vi "ExperimentStateCluster.vi"() -> (2 "Experiment State":T1={"error"={"status"=FALSE, "code"=0, "source"=""}, "Digitizer DAQmx Tasks"={"TaskArray"=[]}, "Digitizer Settings"={"Channel Settings"=[], "Card Settings"=[]}, "Synchronization Settings"={"Synchronizer"="PXI1Slot2", "source terminal"="GlobalSoftwareTrigger"}, "Digitizer Data"=[], "Next Shot#"="0", "System Message"="", "User Shot Notes"="", "Timing Settings"={"Timing Card Settings"=[], "Timing Channel Settings"=[[{"Delay (s)"=2.559999942779541, "Pulse width (s)"=0.009999999776482582, "Active"=TRUE, "Channel Name"="Fiber 8", "counter"="PXI1Slot8/ctr7", "FrontPanelTime"=2.559999942779541}]]}, "Timing Tasks"={"TaskArray"=[]}, "Tree"="0", "Time Card/Channels"=[2, 8], "DAQ Card/Channels"=[3, 8], "Program Version"="", "RIO Settings"={"Channel Settings"=[], "Card Settings"=[]}, "RIO References"={"Reference Array"=[]}} {"RIO Settings"."Card Settings"."Sample Rate" format="%#_3p"; "Timing Settings"."Timing Channel Settings"."FrontPanelTime" format="%.3p"; "Timing Settings"."Timing Channel Settings"."Pulse width (s)" format="%.3p"; "Timing Settings"."Timing Channel Settings"."Delay (s)" format="%.3p"; "Digitizer Settings"."Card Settings"."Global Edge Type" items=["Rising"=10280, "Falling"=10171]; "Digitizer Settings"."Card Settings"."Sample Rate" format="%#_3p"})   [LabVIEW 2014]
uses:
  ExperimentStateCluster.ctl
  DigitizerSettingsChannelSettings.ctl
  DigitizerSettingsCardSettingsArray.ctl
  DigitizerSettingsCardSettings.ctl
  TimingSettings.ctl
  TimingCardSettings.ctl
  TimingChannelSettings.ctl
  RIOSettingsExperimentStateCluster.ctl
  RIOSettingsChannelSettings.ctl
  RIOSettingsCardSettingsArray.ctl
  RIOSettingsCardSettings.ctl
  <vilib>/userdefined/High Color/nirio_resource_hc.ctl
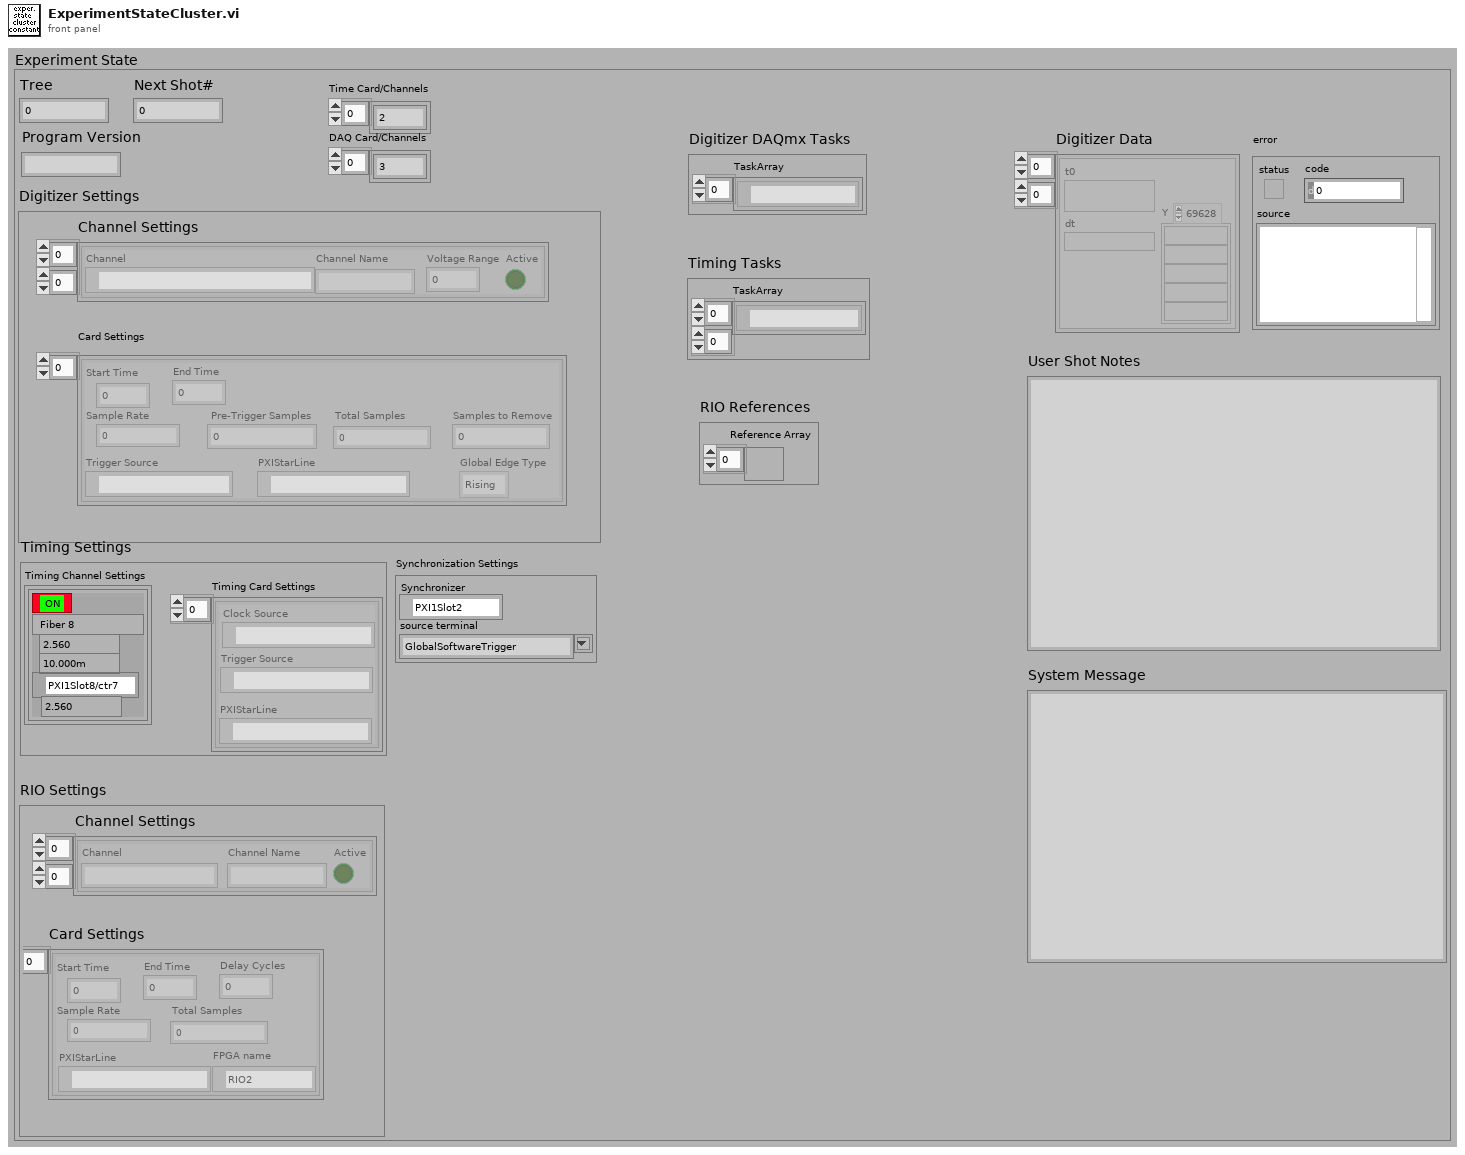
[diagram p1: front panel]
types:
  T1 = typedef "ExperimentStateCluster.ctl" = cluster{"error":errorcluster, "Digitizer DAQmx Tasks":cluster{"TaskArray":refnum<k21>[]}, "Digitizer Settings":cluster{"Channel Settings":T2[][], "Card Settings":T3}, "Synchronization Settings":cluster{"Synchronizer":refnum<k15>, "source terminal":string}, "Digitizer Data":waveform(dbl)[][], "Next Shot#":string, "System Message":string, "User Shot Notes":string, "Timing Settings":T5, "Timing Tasks":cluster{"TaskArray":refnum<k21>[][]}, "Tree":string, "Time Card/Channels":i32[], "DAQ Card/Channels":i32[], "Program Version":string, "RIO Settings":T8, "RIO References":cluster{"Reference Array":refnum<k20>[]}}
  T2 = typedef "DigitizerSettingsChannelSettings.ctl" = cluster{"Channel":tag, "Channel Name":string, "Voltage Range":dbl, "Active":bool}
  T3 = typedef "DigitizerSettingsCardSettingsArray.ctl" = T4[]
  T4 = typedef "DigitizerSettingsCardSettings.ctl" = cluster{"Start Time":dbl, "End Time":dbl, "Sample Rate":dbl, " Pre-Trigger Samples":u32, "Total Samples":i32, "Samples to Remove":u32, "Trigger Source":tag, "Global Edge Type":i32, "PXIStarLine":tag}
  T5 = typedef "TimingSettings.ctl" = cluster{"Timing Card Settings":T6[], "Timing Channel Settings":T7[][]}
  T6 = typedef "TimingCardSettings.ctl" = cluster{"Trigger Source":tag, "Clock Source":tag, "PXIStarLine":tag}
  T7 = typedef "TimingChannelSettings.ctl" = cluster{"Delay (s)":dbl, "Pulse width (s)":dbl, "Active":bool, "Channel Name":string, "counter":tag, "FrontPanelTime":dbl}
  T8 = typedef "RIOSettingsExperimentStateCluster.ctl" = cluster{"Channel Settings":T9[][], "Card Settings":T10}
  T9 = typedef "RIOSettingsChannelSettings.ctl" = cluster{"Channel Name":string, "Active":bool, "Channel":string}
  T10 = typedef "RIOSettingsCardSettingsArray.ctl" = T11[]
  T11 = typedef "RIOSettingsCardSettings.ctl" = cluster{"Start Time":dbl, "End Time":dbl, "Sample Rate":dbl, "Total Samples":u64, "PXIStarLine":tag, "Delay Cycles":u64, "FPGA name":T12}
  T12 = typedef "nirio_resource_hc.ctl" = tag
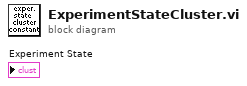
[diagram p0: block diagram]
diagram:
